vi "testing.vi"   [LabVIEW 2016, in "Testing.lvrbt"]
uses:
  Testing.lvrbt
  <vilib>/NXT/Block Support/NXT_InputPort.ctl
  <vilib>/NXT/Block Support/NXT_OutputPort.ctl
  <vilib>/NXT/Dual Mode Library/Sensors/Touch_Pressed.vi
  <vilib>/NXT/NXTIO Xnodes/NXTIONodeSubVIs/NXTMoveMotors.vi
  <vilib>/NXT/Dual Mode Library/Waits/Wait_Num.vi
  <vilib>/NXT/Subs/LVHSConnector.ctl
  <vilib>/NXT/NXTIO Xnodes/AddressXNode/NXTIOAddress.xnode
  <vilib>/NXT/NXTIO Xnodes/NXTIOXNode/NXTIO.xnode
  <vilib>/NXT/LegoClasses/BrickReference/BrickReference.lvclass
types:
  T1 = typedef "NXT_InputPort.ctl" = u32
  T2 = typedef "NXT_OutputPort.ctl" = u8
  T3 = typedef "LVHSConnector.ctl" = refnum<class "BrickReference.lvclass">
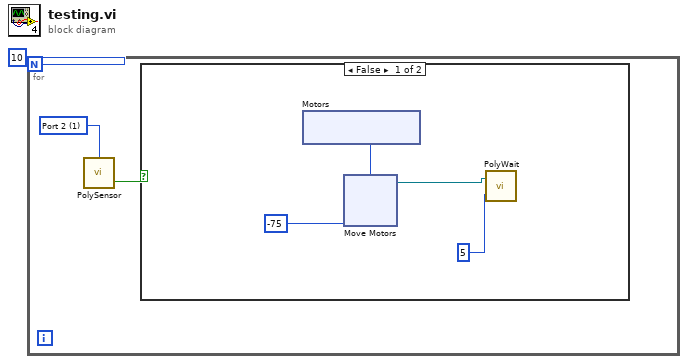
[diagram p0: block diagram]
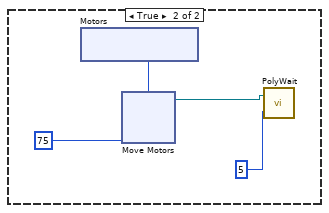
[diagram p2: hidden frame]
diagram:
  n1 = for {
    N: 10 -> [_]
    w3 = T1 1 items=["Port 1", "Port 2", "Port 3", "Port 4"] ("Port (Port 1)")
    n2 = call-poly <vilib>:"PolySensor.vi"("Port (Port 1)"=w3) -> ("Yes / No"=w2:bool)  [unwired: 2 in, 1 out]
    n3 = case shown="False" w2 {
      frame False {
        n4 = xnode "Motors"() -> ("Motor"=w5:T2)
        n5 = xnode "Move Motors"("Power/Speed 1"=-75, "Motors"=w5) -> ("NXT/EV3"=w6:T3)  [unwired: 1 in]
        n6 = call-poly <vilib>:"PolyWait.vi"("Time (1 sec)"=5, "NXT/EV3"=w6) -> ()  [unwired: 2 in, 1 out]
      }
      frame True {
        n7 = xnode "Motors"() -> ("Motor"=w19:T2)
        n8 = xnode "Move Motors"("Power/Speed 1"=75, "Motors"=w19) -> ("NXT/EV3"=w18:T3)  [unwired: 1 in]
        n9 = call-poly <vilib>:"PolyWait.vi"("Time (1 sec)"=5, "NXT/EV3"=w18) -> ()  [unwired: 2 in, 1 out]
      }
    }
  }
